vi "Execute event.vi"(8 "error in (no error)":errorcluster, 9 "Event Data":variant, 10 "Button Event":T1, 11 "Button in":refnum<class "Button.lvclass">) -> (0 "error out":errorcluster, 2 "Value Changed ?":bool, 3 "Button out":refnum<class "Button.lvclass">)   [LabVIEW 2012, in "Button.lvclass"]
doc: "The button method that is actually called when the a button is clicked/latched or unlatched. This is where one would hook an custom actions by overiding this method."
uses:
  Button.lvclass
  Type Defs/Button Events.ctl
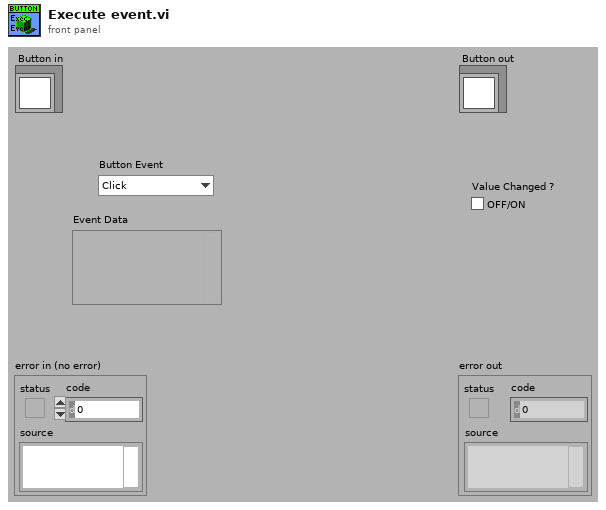
[diagram p1: front panel]
types:
  T1 = typedef "Button.lvclass/Button Events.ctl" = enum16{"Click", "Latch", "Unlatch"}
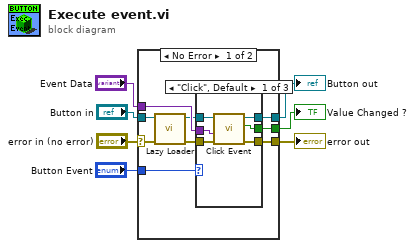
[diagram p0: block diagram]
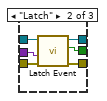
[diagram p2: hidden frame]
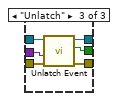
[diagram p3: hidden frame]
diagram:
  n1 = case shown="No Error" "error in (no error)" {
    selector: "error in (no error)" -> [w9 w36]
    tunnel: [w14 w36] -> w6
    tunnel: [w15 w35] -> w4
    tunnel: "Button in" -> [w11 w35]
    tunnel: "Event Data" -> [w13 _]
    tunnel: "Button Event" -> [w16 _]
    tunnel: [w12 _] -> w1
    frame No Error {
      n2 = call "Lazy Loader.vi"("error in (no error)"=w9, "object in"=w11) -> ("error out"=w8:errorcluster, "object out"=w10:refnum<class "Button.lvclass">)  [unwired: 8 in]
      n3 = case shown="\"Click\", Default" w16 {
        tunnel: w10 -> [w22 w28 w34]
        tunnel: [w21 w27 w33] -> w15
        tunnel: w8 -> [w20 w26 w32]
        tunnel: [w19 w25 w31] -> w14
        tunnel: w13 -> [w18 w24 w30]
        tunnel: [w17 w23 w29] -> w12
        frame "Click", Default {
          n4 = call-dynamic "Click Event.vi"("error in (no error)"=w20, "Event Data"=w18, "Button in"=w22) -> ("error out"=w19:errorcluster, "Value Changed ?"=w17:bool, "Button out"=w21:refnum<class "Button.lvclass">)  [unwired: 6 in]
        }
        frame "Latch" {
          n5 = call-dynamic "Latch Event.vi"("error in (no error)"=w26, "Event Data"=w24, "Button in"=w28) -> ("error out"=w25:errorcluster, "Value Changed ?"=w23:bool, "Button out"=w27:refnum<class "Button.lvclass">)  [unwired: 6 in]
        }
        frame "Unlatch" {
          n6 = call-dynamic "Unlatch Event.vi"("error in (no error)"=w32, "Event Data"=w30, "Button in"=w34) -> ("error out"=w31:errorcluster, "Value Changed ?"=w29:bool, "Button out"=w33:refnum<class "Button.lvclass">)  [unwired: 6 in]
        }
      }
    }
    frame Error {
    }
  }
  "error out" <- w6
  "Button out" <- w4
  "Value Changed ?" <- w1
